vi "execute_trajectory.vi"(8 "error in":errorcluster, 10 "File Name":string="path1.path") -> (0 "error out":errorcluster)   [LabVIEW 2020]
doc: "Executes a <i>PathPlanner</i> trajectory file."
uses:
  <vilib>/Rock Robotics/WPI/ThirdParty/JAS_Junk/TrajLib/PID_TUNING.ctl
  <vilib>/Rock Robotics/WPI/ThirdParty/JAS_Junk/TrajLib/ProfiledPIDController_NewPeriod.vi
  <vilib>/Rock Robotics/WPI/ThirdParty/JAS_Junk/TrajLib/ProfiledPIDController_SetIntegratorRange.vi
  <vilib>/Rock Robotics/WPI/ThirdParty/JAS_Junk/TrajLib/ProfiledPIDController_DisableContInput.vi
  <vilib>/Rock Robotics/WPI/ThirdParty/JAS_Junk/TrajLib/ProfiledPIDController_EnableContInput.vi
  <vilib>/Rock Robotics/WPI/ThirdParty/JAS_Junk/TrajLib/TrapProfConstraint_New.vi
  <vilib>/Rock Robotics/WPI/ThirdParty/JAS_Junk/TrajLib/PIDController_NewPeriod.vi
  <vilib>/Rock Robotics/WPI/ThirdParty/JAS_Junk/TrajLib/PIDController_SetIntegratorRange.vi
  <vilib>/Rock Robotics/WPI/ThirdParty/JAS_Junk/TrajLib/PIDController_Reset.vi
  <vilib>/Rock Robotics/WPI/ThirdParty/JAS_Junk/TrajLib/HolDrvCtrl_Calculate.vi
  <vilib>/Rock Robotics/WPI/ThirdParty/JAS_Junk/TrajLib/TrapProfState_New.vi
  <vilib>/Rock Robotics/SystemInterfaces/NetworkCommunication/NetComm_UsageReport_report.vi
  <vilib>/Rock Robotics/WPI/ThirdParty/JAS_Junk/TrajLib/PIDController_DisableContinousInput.vi
  <vilib>/Rock Robotics/WPI/ThirdParty/JAS_Junk/TrajLib/PIDController_EnableContinousInput.vi
  <vilib>/Rock Robotics/WPI/ThirdParty/JAS_Junk/TrajLib/ProfiledPIDController_Calculate_Meas_Goal.vi
  <vilib>/Rock Robotics/WPI/ThirdParty/JAS_Junk/TrajLib/ChassisSpeeds_FromFieldRelativeSpeeds.vi
  <vilib>/Rock Robotics/WPI/ThirdParty/JAS_Junk/TrajLib/PIDController_Calculate_SP_PV.vi
  <vilib>/Rock Robotics/WPI/ThirdParty/JAS_Junk/TrajLib/ProfiledPIDController_Reset_PosOnly.vi
  <vilib>/Rock Robotics/WPI/ThirdParty/JAS_Junk/TrajLib/Pose_getXYAngle.vi
  <vilib>/Rock Robotics/WPI/ThirdParty/JAS_Junk/TrajLib/Rotation_GetAngleCosSin.vi
  <vilib>/Rock Robotics/WPI/ThirdParty/JAS_Junk/TrajLib/Pose_RelativeTo.vi
  <vilib>/Rock Robotics/WPI/ThirdParty/JAS_Junk/TrajLib/Pose_getRotation.vi
  <vilib>/Rock Robotics/WPI/ThirdParty/JAS_Junk/TrajLib/Rotation_Minus.vi
  <vilib>/Rock Robotics/WPI/ThirdParty/JAS_Junk/TrajLib/ProfiledPIDController_SetGoal_PosOnly.vi
  <vilib>/Rock Robotics/WPI/ThirdParty/JAS_Junk/TrajLib/ProfiledPIDController_Calculate_Meas.vi
  <vilib>/Rock Robotics/WPI/ThirdParty/JAS_Junk/TrajLib/Rotation_GetCos.vi
  <vilib>/Rock Robotics/WPI/ThirdParty/JAS_Junk/TrajLib/Rotation_GetSin.vi
  <vilib>/Rock Robotics/WPI/ThirdParty/JAS_Junk/TrajLib/ChassisSpeeds_New.vi
  <vilib>/Rock Robotics/WPI/ThirdParty/JAS_Junk/TrajLib/PIDController_SetSetpoint.vi
  <vilib>/Rock Robotics/WPI/ThirdParty/JAS_Junk/TrajLib/PIDController_Calculate_PV.vi
  <vilib>/Rock Robotics/WPI/ThirdParty/JAS_Junk/TrajLib/ProfiledPIDController_Reset.vi
  <vilib>/Rock Robotics/WPI/ThirdParty/JAS_Junk/TrajLib/Transform_Create_PosePose.vi
  <vilib>/Rock Robotics/WPI/ThirdParty/JAS_Junk/TrajLib/Pose_New_TRRO.vi
  <vilib>/Rock Robotics/WPI/ThirdParty/JAS_Junk/TrajLib/Rotation_UnaryMinus.vi
  <vilib>/Rock Robotics/WPI/ThirdParty/JAS_Junk/TrajLib/Rotation_RotateBy.vi
  <vilib>/Rock Robotics/WPI/ThirdParty/JAS_Junk/TrajLib/ProfiledPIDController_SetGoal.vi
  <vilib>/Rock Robotics/WPI/ThirdParty/JAS_Junk/TrajLib/TrapProfile_New.vi
  <vilib>/Rock Robotics/WPI/ThirdParty/JAS_Junk/TrajLib/ProfiledPIDController_GetPeriod.vi
  <vilib>/Rock Robotics/WPI/ThirdParty/JAS_Junk/TrajLib/TrapProfile_Calculate.vi
  <vilib>/Rock Robotics/WPI/ThirdParty/JAS_Junk/TrajLib/ControllerUtil_GetModulusError.vi
  <vilib>/Rock Robotics/WPI/ThirdParty/JAS_Junk/TrajLib/Translation_RotateBy.vi
  <vilib>/Rock Robotics/WPI/ThirdParty/JAS_Junk/TrajLib/Translation_Minus.vi
  <vilib>/Rock Robotics/WPI/ThirdParty/JAS_Junk/TrajLib/Rotation_CreateXY.vi
  <vilib>/Rock Robotics/WPI/ThirdParty/JAS_Junk/TrajLib/TrapProfile_ShouldFlipAcceleration.vi
  <vilib>/Rock Robotics/WPI/ThirdParty/JAS_Junk/TrajLib/TrapProfile_Direct.vi
  <vilib>/Rock Robotics/WPI/ThirdParty/JAS_Junk/TrajLib/PIDController_GetPeriod.vi
  <vilib>/Rock Robotics/WPI/ThirdParty/JAS_Junk/TrajLib/Translation_Create.vi
  <vilib>/Rock Robotics/WPI/ThirdParty/JAS_Junk/TrajLib/Util_CalcDist.vi
  <vilib>/Utility/semaphor.llb/Obtain Semaphore Reference.vi
  <vilib>/Rock Robotics/WPI/ThirdParty/JAS_Junk/TrajLib/Timer_Reset.vi
  <vilib>/Rock Robotics/WPI/ThirdParty/JAS_Junk/TrajLib/Util_LibraryGlobals.vi
  Subsystems/Swerve/swerve_globals.vi
  <vilib>/Rock Robotics/WPI/ThirdParty/JAS_Junk/TrajLib/Trajectory_Library.lvlib
  <vilib>/Rock Robotics/WPI/ThirdParty/MJansen/PathPlanner/PathPlanner.lvlib
panel:
  in  "Max Accel":dbl=1.58495 format="%20.4f"
  in  "Max Speed":dbl=3.16992 format="%20.4f"
  in  "Theta PID Tuning":T1={"Kp"=0.7, "Ki"=0.0, "Kd"=0.0, "MaximumIntegral"=9.9e+30, "MinimumIntegral"=-9.9e+30}
  in  "XY PID Tuning":T1={"Kp"=5.0, "Ki"=0.0, "Kd"=0.0, "MaximumIntegral"=9.9e+30, "MinimumIntegral"=-9.9e+30}
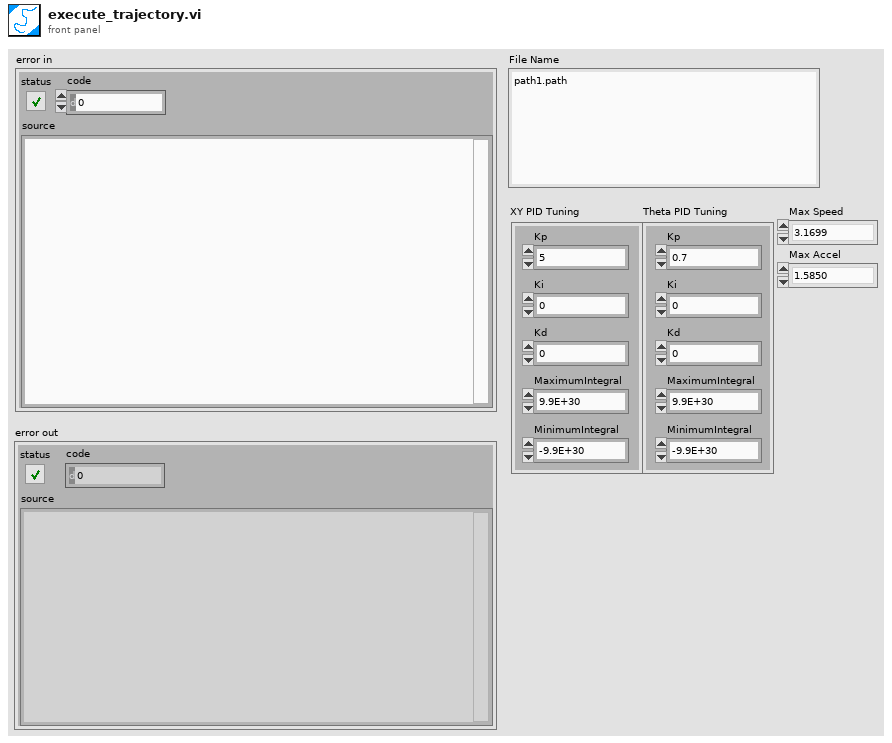
[diagram p1: front panel]
types:
  T1 = typedef "Trajectory_Library.lvlib/PID_TUNING.ctl" = cluster{"Kp":dbl, "Ki":dbl, "Kd":dbl, "MaximumIntegral":dbl, "MinimumIntegral":dbl}
  T2 = typedef "Trajectory_Library.lvlib/PID_CONTROLLER.ctl" = cluster{"Kp":dbl, "Ki":dbl, "Kd":dbl, "Period":dbl, "Max_Integral":dbl, "Min_Integral":dbl, "Max_Input":dbl, "Min_Input":dbl, "Continuous":bool, "PositionError":dbl, "VelocityError":dbl, "PrevError":dbl, "TotalError":dbl, "PositionTolerance":dbl, "VelocityTolerance":dbl, "SetPoint":dbl, "Kf":dbl, "Prev_Deriv":dbl, "Prev_Deriv 2":dbl, "DerivativeFilter":bool, "Min_Output":dbl, "Max_Output":dbl, "Prev_F_P":dbl, "Prev_F_P_2":dbl, "AntiWindupActive":bool, "Measurement":dbl}
  T3 = typedef "Trajectory_Library.lvlib/PROFILED_PID_CONTROLLER.ctl" = cluster{"Controller":T2, "Goal":T4, "Setpoint":T4, "Constraint":T5}
  T4 = typedef "Trajectory_Library.lvlib/TRAPEZOID_PROFILE_STATE.ctl" = cluster{"Position":dbl, "Velocity":dbl}
  T5 = typedef "Trajectory_Library.lvlib/TRAPEZOID_PROFILE_CONSTRAINT.ctl" = cluster{"MaxVelocity":dbl, "MaxAcceleration":dbl}
  T6 = typedef "PathPlanner.lvlib/PathPlannerTrajectory.ctl" = cluster{"TotalTimeSeconds":dbl, "States":T7[]}
  T7 = typedef "PathPlanner.lvlib/PathPlannerState.ctl" = cluster{"AngularAcceleration":T8, "PositionMeters":dbl, "TrajectoryState":T9, "AngularVelocity":T8, "HolonomicRotation":T8, "CurveRadius":dbl, "DeltaPos":dbl}
  T8 = typedef "Trajectory_Library.lvlib/ROTATION2D.ctl" = cluster{"VALUE":dbl, "COS":dbl, "SIN":dbl}
  T9 = typedef "Trajectory_Library.lvlib/TRAJ_STATE.ctl" = cluster{"TimeSeconds":dbl, "Velocity":dbl, "Acceleration":dbl, "POSE":T10, "Curvature":dbl}
  T10 = typedef "Trajectory_Library.lvlib/POSE2D.ctl" = cluster{"TRANSLATION":T11, "ROTATION":T8}
  T11 = typedef "Trajectory_Library.lvlib/TRANSLATION2D.ctl" = cluster{"X":dbl, "Y":dbl}
  T12 = typedef "Trajectory_Library.lvlib/TIMER.ctl" = cluster{"StartTime":dbl, "Accumulated TIme":dbl, "Running":bool, "semaphore":T13}
  T13 = typedef "Semaphore RefNum" = refnum<k1>
  T14 = typedef "Trajectory_Library.lvlib/HOLONOMIC_DRV_CTRL.ctl" = cluster{"poseTolerance":T10, "poseError":T10, "Enabled":bool, "PID_xCtrl":T2, "PID_yCtrl":T2, "PROF_PID_thetaCtrl":T3, "RotationError":T8, "FirstRun":bool}
  T15 = typedef "Trajectory_Library.lvlib/CHASSIS_SPEEDS.ctl" = cluster{"vX":dbl, "vY":dbl, "vOmega":dbl}
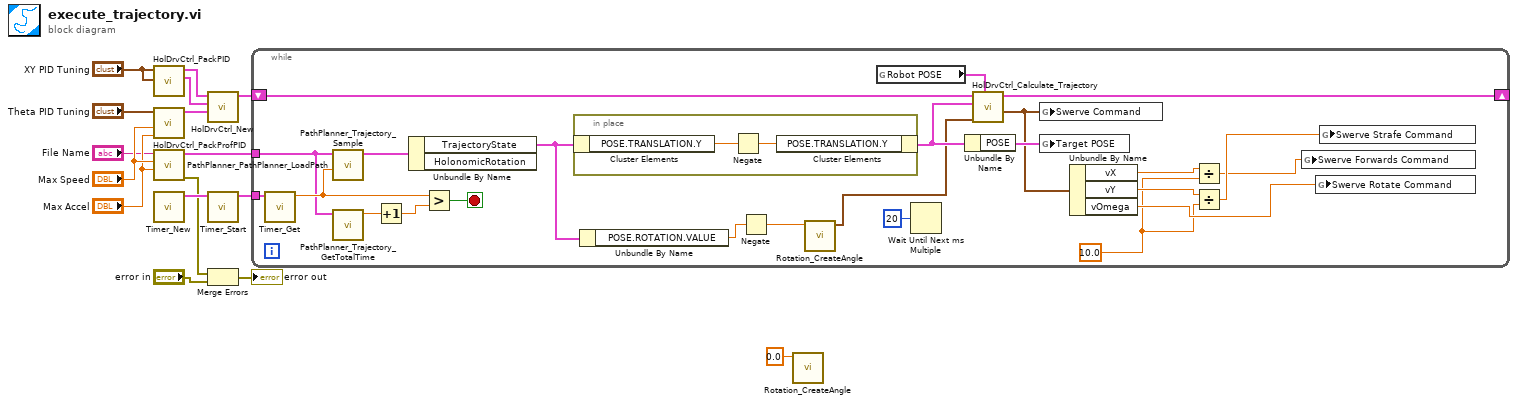
[diagram p0: block diagram]
diagram:
  n1 = call <vilib>:"HolDrvCtrl_PackPID.vi"("Y PID Tuning"="XY PID Tuning", "X PID Tuning"="XY PID Tuning") -> ("Y PID CONTROLLER"=w12:T2, "X PID_CONTROLLER"=w13:T2)  [unwired: 8 in]
  n2 = call <vilib>:"HolDrvCtrl_PackProfPID.vi"("Max Accel"="Max Accel", "Max Speed"="Max Speed", "Theta PID Tuning"="Theta PID Tuning") -> ("Theta PID CONTROLLER"=w15:T3)  [unwired: 8 in]
  n3 = call <vilib>:"PathPlanner_PathPlanner_LoadPath.vi"("MaxAcceleration"="Max Accel", "MaxVelocity"="Max Speed", "FileName"="File Name") -> ("error out"=w6:errorcluster, "PathPlannerTrajectory"=w7:T6)  [unwired: 5 in, 2 out]
  n4 = call <vilib>:"Timer_New.vi"() -> ("TIMER"=w11:T12)  [unwired: 11 in]
  n5 = call <vilib>:"HolDrvCtrl_New.vi"("thetaProfiledPID_CTRL"=w15, "yPID_CTRL"=w12, "xPID_CTRL"=w13) -> ("outHOLONOMIC_DRV_CTRL"=w3:T14)  [unwired: 8 in]
  n6 = call <vilib>:"Timer_Start.vi"("in Timer"=w11) -> ("out Timer"=w2:T12)  [unwired: 10 in]
  n7 = Merge Errors(w6, "error in") -> (→"error out":errorcluster)
  n8 = while {
    tunnel: w2 -> [w40]
    shift-right: [w36] -> _
    shift-left: w3 -> [w37]
    tunnel: w7 -> [w31]
    stop <- w33 stop-if-true
    w22 = 10.0 ("y")
    n9 = call <vilib>:"Timer_Get.vi"("TIMER"=w40) -> ("CurrentTImer"=w32:dbl)  [unwired: 10 in]
    n10 = call <vilib>:"PathPlanner_Trajectory_Sample.vi"("Time"=w32, "PathPlannerTrajectory"=w31) -> ("PathPlannerState"=w39:T7)  [unwired: 9 in]
    n11 = call <vilib>:"PathPlanner_Trajectory_GetTotalTime.vi"("PathPlannerTrajectory"=w31) -> ("TotalTimeSeconds"=w34:dbl)  [unwired: 10 in]
    n12 = Increment(x=w34) -> (x+1=w21:dbl)
    n13 = Unbundle By Name(w39) -> ("TrajectoryState"=w20:T9)  [unwired: 1 out]
    n14 = Greater?(x=w32, y=w21) -> (0:w33:bool)
    n15 = in-place {
      n16 = in-place-cluster #1(w20) -> ("POSE.TRANSLATION.Y"=w42:dbl)
      n17 = Negate(x=w42) -> (-x=w41:dbl)
      n18 = in-place-cluster #1("POSE.TRANSLATION.Y"=w41) -> (w29:T9)
    }
    n19 = Unbundle By Name(w20) -> ("POSE.ROTATION.VALUE"=w19:dbl)
    n20 = Negate(x=w19) -> (-x=w17:dbl)
    n21 = call <vilib>:"Rotation_CreateAngle.vi"("Angle"=w17) -> ("ROTATION"=w18:T8)  [unwired: 10 in]
    n22 = global read "swerve_globals.vi" "Robot POSE"() -> (w38:T10)
    n23 = Wait Until Next ms Multiple(millisecond multiple=u32 20) -> ()  [unwired: 1 out]
    n24 = Unbundle By Name(w29) -> ("POSE"=w30:T10)
    n25 = call <vilib>:"HolDrvCtrl_Calculate_Trajectory.vi"("currentPose"=w38, "angleRef"=w18, "desiredTrajState"=w29, "inHOLONOMIC_DRV_CTRL"=w37) -> ("calcChassisSpeed"=w28:T15, "outHOLONOMIC_DRV_CTRL"=w36:T14)  [unwired: 6 in]
    n26 = global write "swerve_globals.vi" "Swerve Command"(w28) -> ()
    n27 = global write "swerve_globals.vi" "Target POSE"(w30) -> ()
    n28 = Unbundle By Name(w28) -> ("vX"=w27:dbl, "vY"=w26:dbl, "vOmega"=w23:dbl)
    n29 = Divide(x=w27, y=w22) -> (x/y=w24:dbl)
    n30 = Divide(x=w26, y=w22) -> (x/y=w25:dbl)
    n31 = global write "swerve_globals.vi" "Swerve Forwards Command"(w24) -> ()
    n32 = global write "swerve_globals.vi" "Swerve Rotate Command"(w23) -> ()
    n33 = global write "swerve_globals.vi" "Swerve Strafe Command"(w25) -> ()
  }
  n34 = call <vilib>:"Rotation_CreateAngle.vi"("Angle"=0.0) -> ()  [unwired: 10 in, 1 out]
